vi "Keithley DMM7510 Acquire Single.vi"() -> ()   [LabVIEW 2016]
doc: "This example shows how to configure a measurement and take a reading."
uses:
  Keithley DMM7510.lvlib
panel:
  in  "Function":u16(ring) items=["Voltage: DC", "Voltage: AC", "Current: DC", "Current: AC", "2W Resistance", "4W Resistance", "Diode", "Capacitance", "Temperature", "Continuity", "Frequency", "Period", "Ratio", "Digitize Voltage", "Digitize Current"]
  out "Measurement":dbl
  in  "VISA resource name":refnum<visa-resource-name>
  # "(c) 2015 Keithley Instruments,  ALL RIGHTS RESERVED."
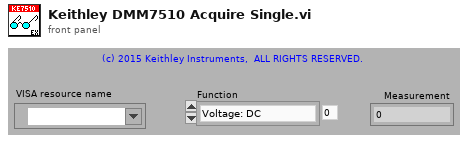
[diagram p1: front panel]
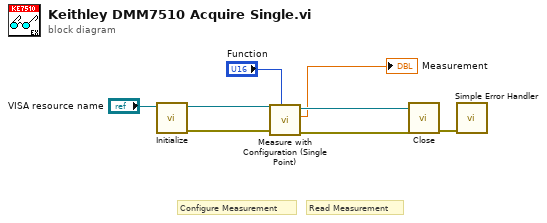
[diagram p0: block diagram]
diagram:
  # "Read Measurement"
  # "Configure Measurement"
  n1 = call "Initialize.vi"("VISA resource name"="VISA resource name") -> ("error out"=w1:errorcluster, "VISA resource name out"=w6:refnum<visa-resource-name>)  [unwired: 9 in]
  n2 = call "Measure with Configuration (Single Point).vi"("Function"="Function", "error in (no error)"=w1, "VISA resource name"=w6) -> ("error out"=w4:errorcluster, "Measurement"=→"Measurement":dbl, "VISA resource name out"=w5:refnum<visa-resource-name>)  [unwired: 5 in, 1 out]
  n3 = call "Close.vi"("error in (no error)"=w4, "VISA resource name"=w5) -> ("error out"=w8:errorcluster)  [unwired: 9 in]
  n4 = call <vilib>:"Simple Error Handler.vi"("error in (no error)"=w8) -> ()  [unwired: 4 in, 5 out]
